vi "Delete1Line.vi"(10 "Value":string) -> (2 "String":string)   [LabVIEW 2017]
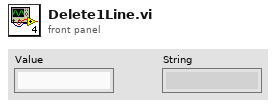
[diagram p1: front panel]
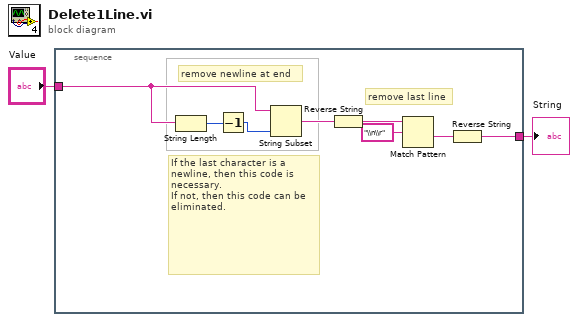
[diagram p0: block diagram]
diagram:
  n1 = stacked-sequence {
    tunnel: "Value" -> [w5]
    tunnel: [w4] -> w2
    frame #0 {
      # "remove last line"
      # "remove newline at end"
      # "If the last character is a newline, then this code is necessary.\nIf not, then this code can be eliminated."
      n2 = String Length(string=w5) -> (length=w8:i32)
      n3 = Decrement(x=w8) -> (x-1=w10:i32)
      n4 = String Subset(string=w5, length (rest)=w10) -> (substring=w9:string)  [unwired: 1 in]
      n5 = Reverse String(1:w9) -> (0:w6:string)
      n6 = Match Pattern(string=w6, regular expression="\\n\\r") -> (after substring=w7:string)  [unwired: 1 in, 3 out]
      n7 = Reverse String(1:w7) -> (0:w4:string)
    }
  }
  "String" <- w2
